vi "grabberpidinit.vi"(9 "setpoint":dbl format="%.2f", 11 "reinitialize? (F) 2":bool) -> (0 "Done? 2":bool)   [LabVIEW 2013]
uses:
  <vilib>/addons/control/pid/pid.llb/PID (DBL).vi
  <vilib>/addons/control/pid/NI_PID_pid.lvlib
panel:
  in  "adjuster":dbl
  in  "PID Gains for Raising/Lowering":T1={"proportional gain (Kc)"=1.2, "integral time (Ti, min)"=0.011, "derivative time (Td, min)"=0.007} {"derivative time (Td, min)" format="%.3f"; "integral time (Ti, min)" format="%.3f"; "proportional gain (Kc)" format="%.3f"}
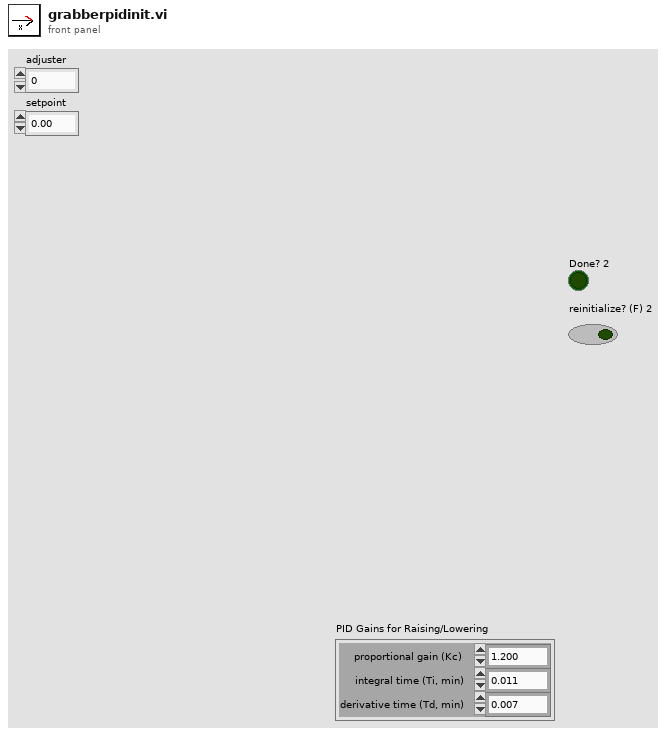
[diagram p1: front panel]
types:
  T1 = cluster{"proportional gain (Kc)":dbl, "integral time (Ti, min)":dbl, "derivative time (Td, min)":dbl}
  T2 = typedef "WPI_EncoderDevRef.ctl" = cluster{"DevStatus":errorcluster, "EncoderIndex":T3, "CounterIndex":T4, "DistancePerCount":dbl, "Decoding Type":T5}
  T3 = typedef "FPGA_EncoderIdx.ctl" = enum8{"Enc 0", "Enc 1", "Enc 2", "Enc 3", "Invalid"}
  T4 = typedef "FPGA_CounterCtrSystemIndex.ctl" = enum8{"Ctr 0", "Ctr 1", "Ctr 2", "Ctr 3", "Ctr 4", "Ctr 5", "Ctr 6", "Ctr 7", "Invalid"}
  T5 = typedef "WPI_EncoderType.ctl" = enum16{"1x", "2x", "4x"}
  T6 = typedef "WPI_DigitalInputDevRef.ctl" = cluster{"DevStatus":errorcluster, "DIO Channel":T7, "Digital Module":T8}
  T7 = typedef "FPGA_DIOChannel.ctl" = enum8{"DIO 1", "DIO 2", "DIO 3", "DIO 4", "DIO 5", "DIO 6", "DIO 7", "DIO 8", "DIO 9", "DIO 10", "DIO 11", "DIO 12", "DIO 13", "DIO 14", "Invalid"}
  T8 = typedef "FPGA_TypedefDigitalModule.ctl" = enum16{"Digital Module 1", "Digital Module 2"}
  T9 = typedef "WPI_MotorControlDeviceRef.ctl" = cluster{"DeviceStatus":errorcluster, "Type":enum16{"PWM", "CAN"}, "PWM":cluster{"Digital Module":T8, "PWM Channel":T10, "DeadBand":T11}, "CAN":cluster{"Device Number":u8, "Control Mode":T12, "Semaphore":T13, "Max Vout":dbl}, "Invert":bool, "TransformRef":T14, "InvTransformRef":T14}
  T10 = typedef "FPGA_DIOPWMChannel.ctl" = enum8{"PWM 1", "PWM 2", "PWM 3", "PWM 4", "PWM 5", "PWM 6", "PWM 7", "PWM 8", "PWM 9", "PWM 10", "Invalid"}
  T11 = typedef "WPI_PWMDeadband.ctl" = cluster{"Name":string, "maxPositivePwm":i32, "minPositivePwm":i32, "centerPwm":i32, "maxNegativePwm":i32, "minNegativePwm":i32, "angularRange":u16}
  T12 = typedef "WPI_CANJaguar_ControlMode.ctl" = enum8{"Percent VBus", "Current", "Speed", "Position", "Voltage"}
  T13 = typedef "Semaphore RefNum" = refnum<k1>
  T14 = typedef "WPI_PWMTransform_ConPane.ctl" = refnum<vi>
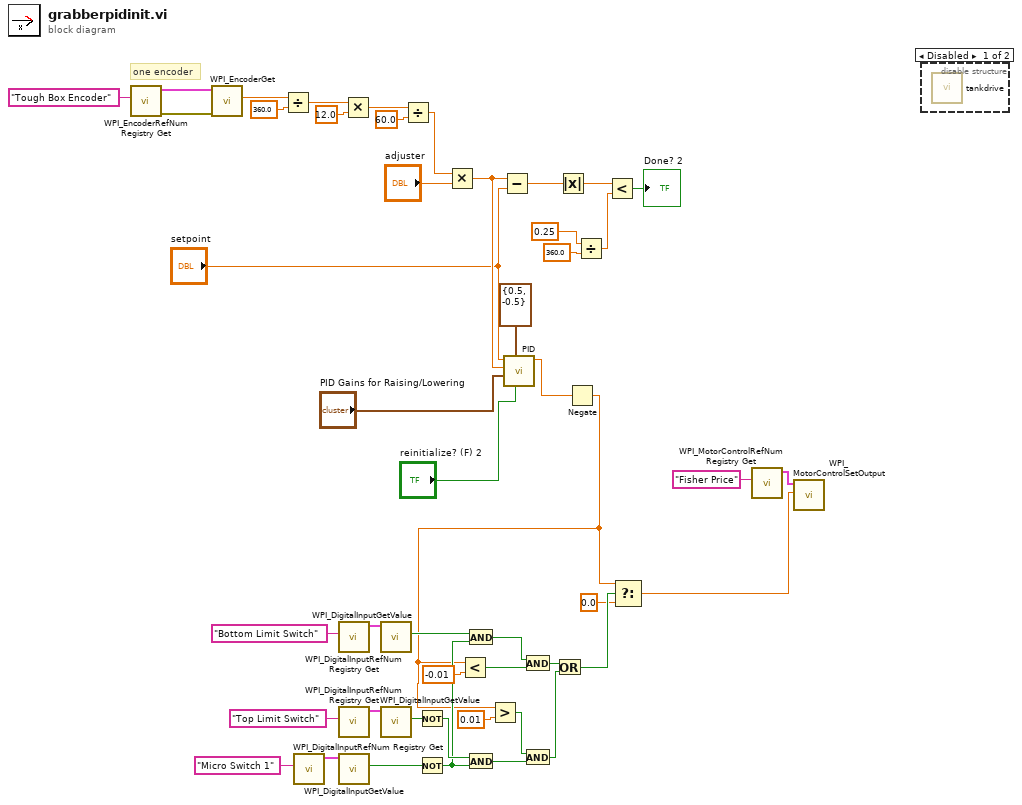
[diagram p0: block diagram]
diagram:
  # "one encoder"
  n1 = call <vilib>:"WPI_EncoderRefNum Registry Get.vi"("refnum name"="Tough Box Encoder") -> ("error out"=w48:errorcluster, "EncoderDevRef"=w47:T2)  [unwired: 9 in]
  n2 = call <vilib>:"WPI_EncoderGet.vi"("error in (no error)"=w48, "EncoderDevRef"=w47) -> ("Distance"=w38:dbl)  [unwired: 4 in, 5 out]
  n3 = Divide(x=w38, y=360.0) -> (x/y=w36:dbl)
  n4 = call <vilib>:"WPI_DigitalInputRefNum Registry Get.vi"("refnum name"="Micro Switch 1") -> ("DigitalInputDevRef"=w18:T6)  [unwired: 9 in, 1 out]
  n5 = call <vilib>:"WPI_DigitalInputRefNum Registry Get.vi"("refnum name"="Bottom Limit Switch") -> ("DigitalInputDevRef"=w22:T6)  [unwired: 9 in, 1 out]
  n6 = call <vilib>:"WPI_DigitalInputRefNum Registry Get.vi"("refnum name"="Top Limit Switch") -> ("DigitalInputDevRef"=w13:T6)  [unwired: 9 in, 1 out]
  n7 = call <vilib>:"WPI_DigitalInputGetValue.vi"("DigitalInputDevRef"=w18) -> ("Value"=w19:bool)  [unwired: 8 in, 2 out]
  n8 = Multiply(x=w36, y=12.0) -> (x*y=w37:dbl)
  n9 = call <vilib>:"WPI_DigitalInputGetValue.vi"("DigitalInputDevRef"=w22) -> ("Value"=w8:bool)  [unwired: 8 in, 2 out]
  n10 = call <vilib>:"WPI_DigitalInputGetValue.vi"("DigitalInputDevRef"=w13) -> ("Value"=w15:bool)  [unwired: 8 in, 2 out]
  n11 = Divide(x=w37, y=60.0) -> (x/y=w33:dbl)
  n12 = Not(x=w15) -> (.not. x?=w16:bool)
  n13 = Not(x=w19) -> (.not. x?=w7:bool)
  n14 = Multiply(x=w33, y="adjuster") -> (x*y=w31:dbl)
  n15 = And(x=w8, y=w7) -> (x .and. y?=w6:bool)
  n16 = And(x=w16, y=w7) -> (x .and. y?=w11:bool)
  n17 = Subtract(x=w31, y="setpoint") -> (x-y=w43:dbl)
  n18 = call-poly <vilib>:"PID.vi"("reinitialize? (F)"="reinitialize? (F) 2", "output range"=cluster{"output high":dbl, "output low":dbl} {"output high"=0.5, "output low"=-0.5}, "PID gains"="PID Gains for Raising/Lowering", "process variable"=w31, "setpoint"="setpoint") -> ("output"=w5:dbl)  [unwired: 5 in, 1 out]
  n19 = Absolute Value(x=w43) -> (abs(x)=w44:dbl)
  n20 = Negate(x=w5) -> (-x=w3:dbl)
  n21 = Less?(x=w3, y=-0.01) -> (x < y?=w21:bool)
  n22 = Greater?(x=w3, y=0.01) -> (0:w12:bool)
  n23 = And(x=w6, y=w21) -> (x .and. y?=w9:bool)
  n24 = And(x=w12, y=w11) -> (x .and. y?=w10:bool)
  n25 = Or(x=w9, y=w10) -> (x .or. y?=w4:bool)
  n26 = Divide(x=0.25, y=360.0) -> (x/y=w27:dbl)
  n27 = Less?(x=w44, y=w27) -> (x < y?=→"Done? 2":bool)
  n28 = Select(t=w3, s=w4, f=0.0) -> (s? t:f=w2:dbl)
  n29 = call <vilib>:"WPI_MotorControlRefNum Registry Get.vi"("refnum name"="Fisher Price") -> ("MotorControlDevRef"=w25:T9)  [unwired: 9 in, 1 out]
  n30 = call <vilib>:"WPI_MotorControlSetOutput.vi"("Output"=w2, "MotorControlDevRef"=w25) -> ()  [unwired: 7 in, 3 out]
  n31 = disable-structure shown="Disabled" {
    frame Disabled {
      n32 = call "tankdrive.vi"() -> ()  [unwired: 12 in]
    }
    frame Enabled {
    }
  }
